vi "Read Exposure Time.vi"(8 "error in (no error)":errorcluster, 11 "CCDCamera in":refnum<class "CCDCamera.lvclass">) -> (0 "error out":errorcluster, 2 "Exposure Time":sgl format="%.2f", 3 "CCDCamera out":refnum<class "CCDCamera.lvclass">)   [LabVIEW 2018, in "CCDCamera.lvclass"]
uses:
  CCDCamera.lvclass
  CCDCamera.lvclass/CCDCamera.ctl
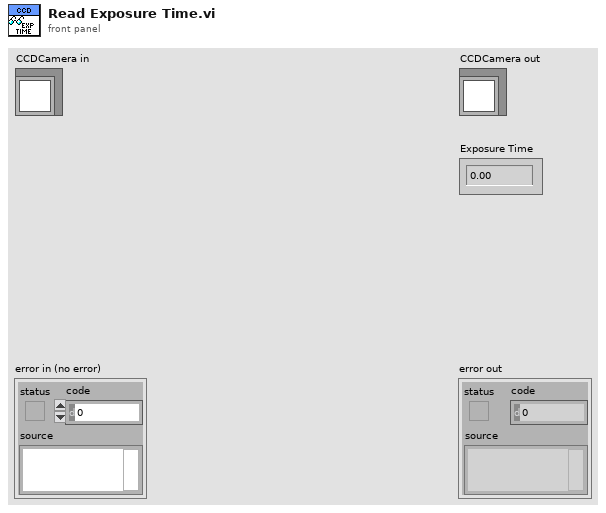
[diagram p1: front panel]
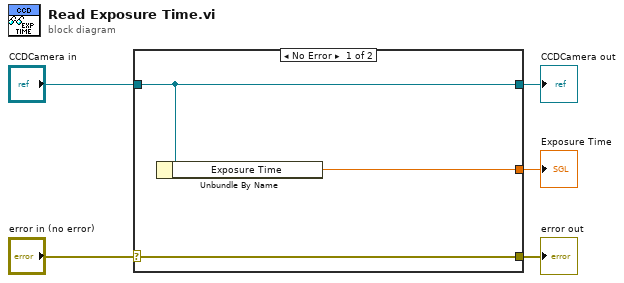
[diagram p0: block diagram]
diagram:
  n1 = case shown="No Error" "error in (no error)" {
    selector: "error in (no error)" -> [w8 w9]
    tunnel: [w8 w9] -> w4
    tunnel: [w7 w10] -> w2
    tunnel: "CCDCamera in" -> [w7 w10]
    tunnel: [w6 _] -> w1
    frame No Error {
      n2 = Unbundle By Name(w7) -> ("Exposure Time"=w6:sgl)
    }
    frame Error {
    }
  }
  "error out" <- w4
  "CCDCamera out" <- w2
  "Exposure Time" <- w1
